vi "3D Graph.vi"() -> ()   [LabVIEW 2013]
panel:
  out "Legend":refnum<vi>(3d-picture)
  in  "Target Theta":sgl
  in  "Target Phi":sgl
  in  "Target Magnitude":sgl=1.0
  in  "Field Theta":sgl
  in  "Field Phi":sgl
  in  "Field Magnitude":sgl=1.0
  out "3D Picture":refnum<vi>(3d-picture)
  # "x = red\ny = green\nz - blue"
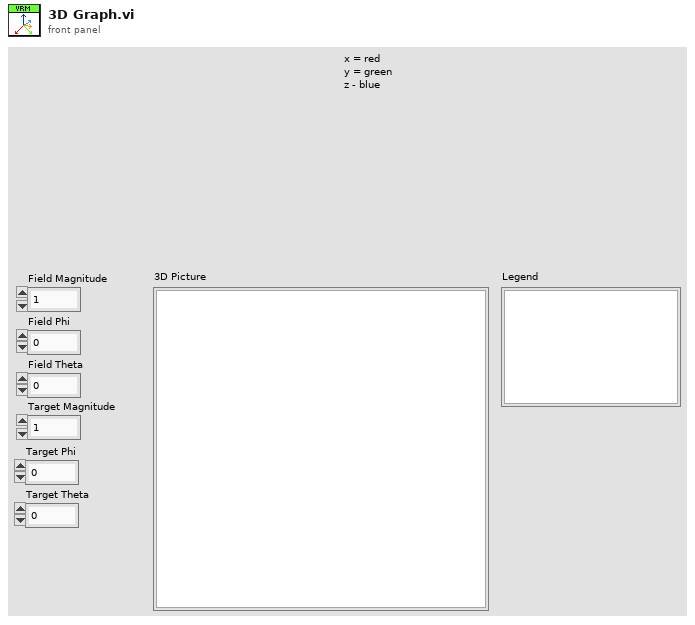
[diagram p1: front panel]
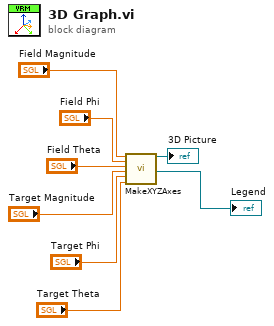
[diagram p0: block diagram]
diagram:
  n1 = call "MakeXYZAxes.vi"("Field Magnitude"="Field Magnitude", "Field Phi"="Field Phi", "Field Theta"="Field Theta", "Target Magnitude"="Target Magnitude", "Target Phi"="Target Phi", "Target Theta"="Target Theta") -> ("Field Graph"=→"3D Picture":refnum<vi>, "Legend"=→"Legend":refnum<vi>)  [unwired: 11 in, 1 out]
